vi "System shutdown.vi"(8 "error in (no error)":errorcluster, 11 "Guardian in":refnum<class "Guardian.lvclass">) -> (0 "error out":errorcluster, 3 "Guardian out":refnum<class "Guardian.lvclass">)   [LabVIEW 2026, in "TALOS.lvlib" / "Guardian.lvlib" / "Guardian.lvclass"]
uses:
  Guardian.lvclass
  C:/LabVIEW Code/TALOS/builds/Actor Framework PPL/Actor Framework.lvlibp/1abvi3w/vi.lib/ActorFramework/Actor/Actor.lvclass
  Classes/uService List/uService List.lvclass/uService List.ctl
  builds/Actor Framework PPL/Actor Framework.lvlibp/1abvi3w/vi.lib/ActorFramework/Message Enqueuer/Message Priority.ctl
  Father of all uServices/Father of all uServices/Event Handler Items.ctl
  Father of all uServices/Father of all uServices Messages/Event Handler Msg/Event Handler Msg.lvclass/Event Handler Msg.ctl
  Ancestor/Ancestor/Ancestor.lvclass/Ancestor.ctl
  Classes/uService List/Get all Queue.vi
  c098ac5f-852a-42ba-a463-646f2b06a1c5.vi
  Support VIs/Generate Error.vi
  FGV/Error Memory/Get Error Description.vi
  Support VIs/Get PC name.vi
  Ancestor/Ancestor/Read ID.vi
  Support VIs/Get Class Name.vi
  <vilib>/Utility/error.llb/Clear Errors.vi
  FGV/Error Memory/Error Memory Core.vi
  <vilib>/AdvancedString/Delimited String to 1D String Array.vi
  <vilib>/AdvancedString/Delimited String to 1D String Array (string).vi
  Support VIs/Circus Root Path.vi
  FGV/Error Memory/Error Crt Lvl checker.vi
  FGV/Error Memory/Error Memory Core.vi/40c8088d-b597-4017-91af-faa98e00292e.vi
  FGV/Error Memory/Error Memory Core.vi/d4a3ab98-063c-4e44-b43d-fbdcfe6c2be2.vi
  builds/Actor Framework PPL/Actor Framework.lvlibp/1abvi3w/vi.lib/ActorFramework/Message Enqueuer/Enqueue.vi
  Support VIs/Global Memory.vi
  <vilib>/Utility/LVClass/Get LV Class Name.vi
  Support VIs/Is in Packed Library.vi
  Support VIs/TALOS Root path.vi
  Support VIs/Read CSV worksheet.vi
  Support VIs/Global Constants.vi
  <vilib>/Utility/error.llb/General Error Handler.vi
  Support VIs/Error Log.vi
  Father of all uServices/Father of all uServices Messages/Event Handler Msg/Event Handler Msg.lvclass
  Ancestor/Ancestor/Ancestor.lvclass
  <vilib>/Comparison/Equal/Equal Functor/Equal Functor.lvclass
  builds/Actor Framework PPL/Actor Framework.lvlibp/1abvi3w/vi.lib/ActorFramework/Actor/Actor.lvclass
  builds/Actor Framework PPL/Actor Framework.lvlibp/1abvi3w/vi.lib/ActorFramework/Stop Msg/Stop Msg.lvclass
  Classes/uService List/uService List.lvclass
  builds/Actor Framework PPL/Actor Framework.lvlibp/1abvi3w/vi.lib/ActorFramework/Message Enqueuer/Message Enqueuer.lvclass
  Father of all uServices/Father of all uServices/Father of all uServices.lvclass
  TALOS.lvlib
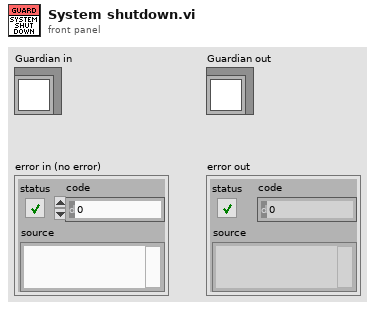
[diagram p1: front panel]
types:
  T1 = typedef "TALOS.lvlib/Father of all uServices.lvlib/Father of all uServices.lvclass/Event Handler Items.ctl" = enum16{"Button Pressed", "Message", "Ready to launch?", "Safe Mode", "Start RUN", "Stop RUN"}
  T2 = typedef "Actor Framework.lvlibp/Message Enqueuer.lvclass/Message Priority.ctl" = enum16{"Low", "Normal", "High"}
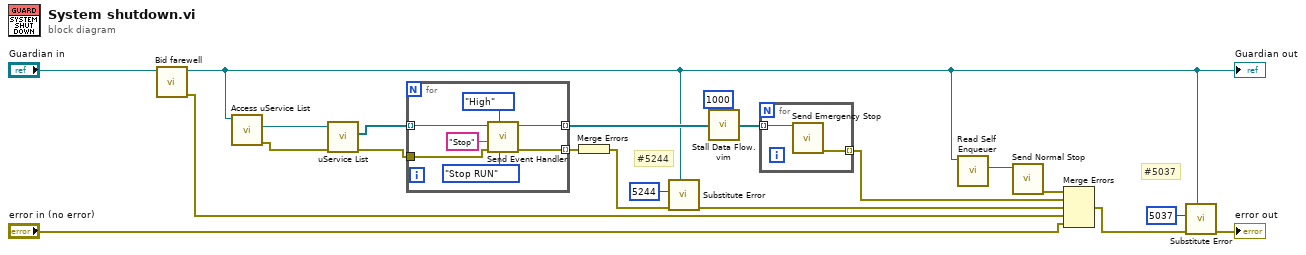
[diagram p0: block diagram]
diagram:
  # "#5037"
  # "#5244"
  n1 = call "Bid farewell.vi"("Guardian in"="Guardian in") -> ("error out"=w1:errorcluster, "Guardian out"=w3:refnum<class "Guardian.lvclass">)  [unwired: 9 in]
  "Guardian out" <- w3
  n2 = call-dynamic "Access uService List.vi"("Ancestor in"=w3) -> ("error out"=w12:errorcluster, "uService List out"=w19:refnum<class "uService List.lvclass">)  [unwired: 8 in, 1 out]
  n3 = call-poly "uService List.vi"("error in (no error)"=w12, "uService List"=w19) -> ("error out"=w11:errorcluster, "All queues"=w18:refnum<class "Message Enqueuer.lvclass">[])  [unwired: 7 in, 1 out]
  n4 = for {
    tunnel: w18 -> [w28] mode=indexing
    tunnel: [w25] -> w13 mode=indexing
    tunnel: [w23] -> w15 mode=indexing
    tunnel: w11 -> [w22]
    n5 = call "Send Event Handler.vi"("Event type"=Event_Handler_Items."Stop RUN", "Message Priority (Normal)"=Message_Priority."High", "error in (no error)"=w22, "Item Name"="Stop", "Message Enqueuer"=w28) -> ("error out"=w25:errorcluster, "Message Enqueuer out"=w23:refnum<class "Message Enqueuer.lvclass">)  [unwired: 5 in]
  }
  n6 = Merge Errors(w13) -> (w10:errorcluster)
  n7 = call "Substitute Error.vi"("LabVIEW Object"=w3, "error in (no error)"=w10, "Error Code"=5244) -> ("error out"=w9:errorcluster)  [unwired: 8 in]
  n8 = call "Stall Data Flow.vim"("value in"=w15, "milliseconds to wait"=u32 1000) -> ("value out"=w14:refnum<class "Message Enqueuer.lvclass">[])  [unwired: 1 out]
  n9 = for {
    tunnel: w14 -> [w30] mode=indexing
    tunnel: [w29] -> w17 mode=indexing
    n10 = call "Send Emergency Stop.vi"("Message Enqueuer"=w30) -> ("error out"=w29:errorcluster)  [unwired: 10 in]
  }
  n11 = call "Read Self Enqueuer.vi"("Actor"=w3) -> ("Self Enqueuer"=w20:refnum<class "Message Enqueuer.lvclass">)  [unwired: 10 in]
  n12 = call "Send Normal Stop.vi"("Message Enqueuer"=w20) -> ("error out"=w21:errorcluster)  [unwired: 10 in]
  n13 = Merge Errors(w21, w17, w9, w1, "error in (no error)") -> (w7:errorcluster)
  n14 = call "Substitute Error.vi"("LabVIEW Object"=w3, "error in (no error)"=w7, "Error Code"=5037) -> ("error out"=→"error out":errorcluster)  [unwired: 8 in]
